vi "Release Session.vi"(0 "Session Handle":T1, 11 "error in (no error)":errorcluster, 13 "force destroy? (F)":bool) -> (15 "error out":errorcluster)   [LabVIEW 2018, in "Test Number and Bin Generator.lvlib" / "Test Number and Bin Generator.lvclass"]
doc: "Releases an obtained reference to the session"
uses:
  Test Number and Bin Generator.lvclass
  Typedefs/Session Handle.ctl
  C:/Sequence Automation/Plugins/Sequence Automation Session.lvlibp/Sequence Automation Session.lvclass
  Plugins/Sequence Automation Session.lvlibp/Sequence Automation Session.lvclass
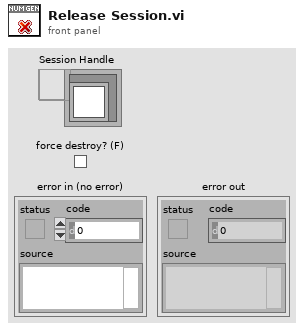
[diagram p1: front panel]
types:
  T1 = typedef "Test Number and Bin Generator.lvlib/Test Number and Bin Generator.lvclass/Session Handle.ctl" = refnum<data-value>
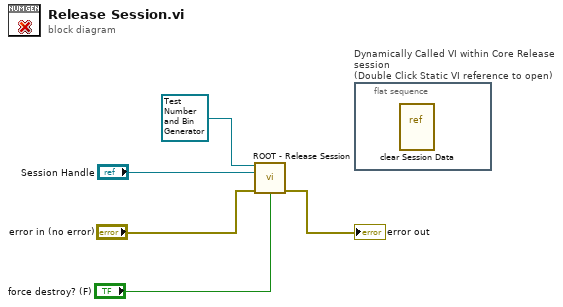
[diagram p0: block diagram]
diagram:
  n1 = call "ROOT - Release Session.vi"("OBJ - Session in"=refnum<class "Test Number and Bin Generator.lvclass"> refnum ("Test Number and Bin Generator.lvlib:Test Number and Bin Generator"), "Session Handle in"="Session Handle", "error in (no error)"="error in (no error)", "force destroy? (F)"="force destroy? (F)") -> ("error out"=→"error out":errorcluster)  [unwired: 10 in, 1 out]
  n2 = flat-sequence "Dynamically Called VI within Core Release session\n(Double Click Static VI reference to open)" {
    frame #0 {
      n3 = vi-ref "clear Session Data.vi"() -> ()  [unwired: 1 out]
    }
  }
